vi "Load PQ .ptu FLI Dataset Prelude.vi"(8 "error in (no error)":errorcluster, 11 "File Path in":path) -> (0 "error out":errorcluster, 1 "Metadata":string, 2 "FLI Data File Information":T1, 3 "File Path out":path, 4 "Data Description":string)   [LabVIEW 2021, in "PicoQuant.lvlib"]
uses:
  PicoQuant.lvlib
  AlliGator/AlliGator FLI Data File Information.ctl
  Phasor/Phasor Fluorescence Lifetime Parameters v3.ctl
  AlliGator/AlliGator FLI Dataset Type.ctl
  AlliGator/AlliGator Files.lvlib
  AlliGator/AlliGator HDF5.lvlib
  Phasor/Phasor.lvlib
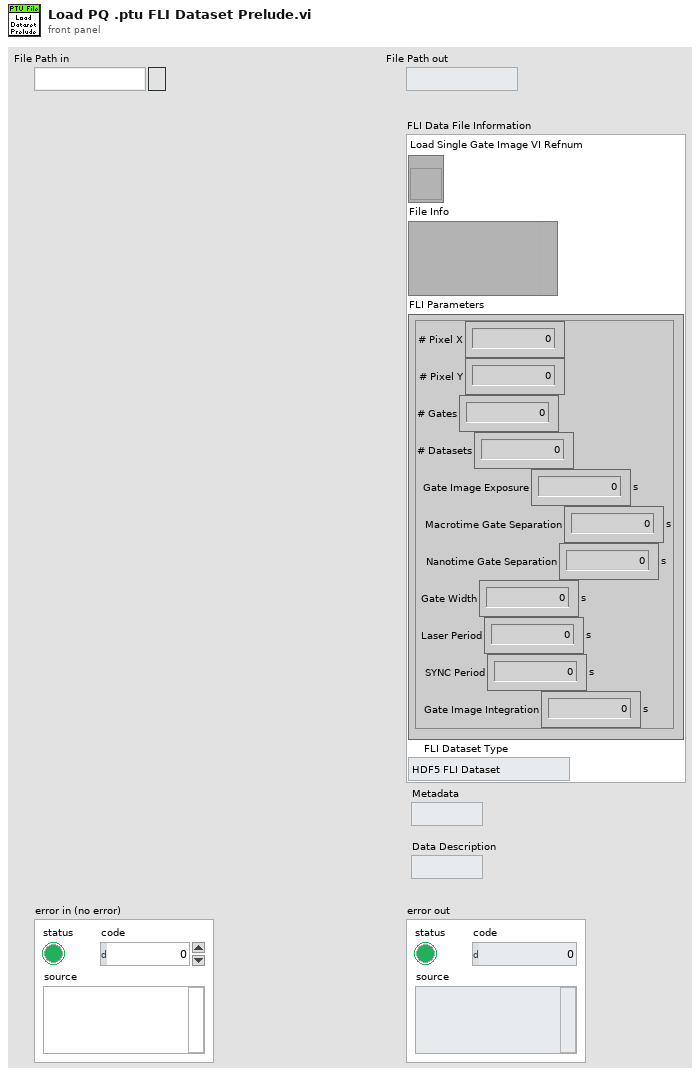
[diagram p1: front panel]
types:
  T1 = typedef "AlliGator HDF5.lvlib/AlliGator FLI Data File Information.ctl" = cluster{"Load Single Gate Image VI Refnum":refnum<vi>, "File Info":variant, "FLI Parameters":T2, "FLI Dataset Type":T3}
  T2 = typedef "Phasor.lvlib/Phasor Fluorescence Lifetime Parameters v3.ctl" = cluster{"# Pixel X":i32, "# Pixel Y":i32, "# Gates":i32, "# Datasets":i32, "Gate Image Exposure":dbl[unit], "Macrotime Gate Separation":dbl[unit], "Nanotime Gate Separation":dbl[unit], "Gate Width":dbl[unit], "Laser Period":dbl[unit], "SYNC Period":dbl[unit], "Gate Image Integration":dbl[unit]}
  T3 = typedef "AlliGator Files.lvlib/AlliGator FLI Dataset Type.ctl" = enum16{"HDF5 FLI Dataset", "Gate Image Folder", ".sdt FLI Dataset (Becker & Hickl)", ".ptu FLI Dataset (PicoQuant)", "SS1 FLI Dataset", "SS2 FLI Dataset", "I/m/phi Dataset", ".bin FLI Dataset (PicoQuant Binned)", ".bin FLI Dataset (Piccolo Binned)"}
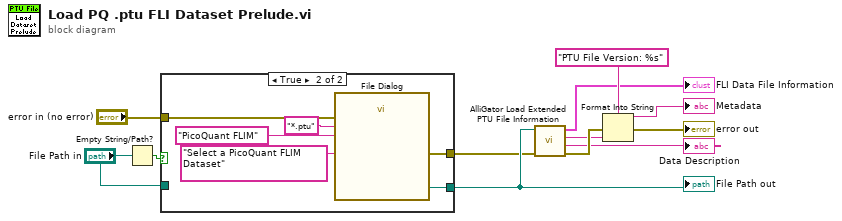
[diagram p0: block diagram]
diagram:
  n1 = Empty String/Path?(string/path="File Path in") -> (empty?=w3:bool)
  n2 = case shown="True" w3 {
    tunnel: "error in (no error)" -> [w13 w20]
    tunnel: [w14 w16] -> w5
    tunnel: [w13 w15] -> w4
    tunnel: "File Path in" -> [w14 _]
    frame False {
    }
    frame True {
      n3 = call "File Dialog"("prompt"="Select a PicoQuant FLIM Dataset", "error in"=w20, "pattern (all files)"="*.ptu", "pattern label"="PicoQuant FLIM") -> ("selected path"=w16:path, "error out"=w15:errorcluster)  [unwired: 8 in, 2 out]
    }
  }
  "File Path out" <- w5
  n4 = call "AlliGator Load Extended PTU File Information.vi"("Error In"=w4, "File Path"=w5) -> ("Error Out"=w10:errorcluster, "Data Description"=→"Data Description":string, "Version"=w9:string, "FLI Data File Information"=→"FLI Data File Information":T1)  [unwired: 3 in, 3 out]
  n5 = Format Into String(format string="PTU File Version: %s", error in=w10, w9) -> (resulting string=→"Metadata":string, error out=→"error out":errorcluster)  [unwired: 1 in]
